vi "GetDeviceSubsetForDeployment.vi"(7 "num":i32=2, 8 "error in (no error)":errorcluster, 9 "i":i32, 10 "DeviceList":T1[](array[typedef])) -> (0 "Error Out":errorcluster, 2 "subarray":T1[](array[typedef]))   [LabVIEW 2016]
uses:
  <vilib>/addons/InsightCM/MessageBus/MessageLibrary/SysCfgDeployer/controls/SysCfgDeployPackageRequestBody.ctl
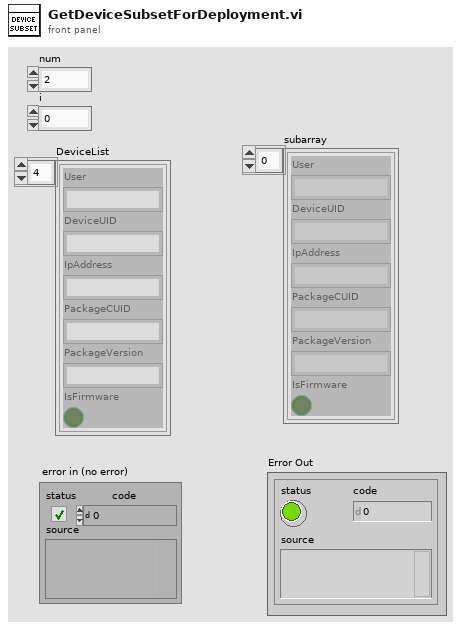
[diagram p1: front panel]
types:
  T1 = typedef "SysCfgDeployPackageRequestBody.ctl" = cluster{"User":string, "DeviceUID":string, "IpAddress":string, "PackageCUID":string, "PackageVersion":string, "IsFirmware":bool}
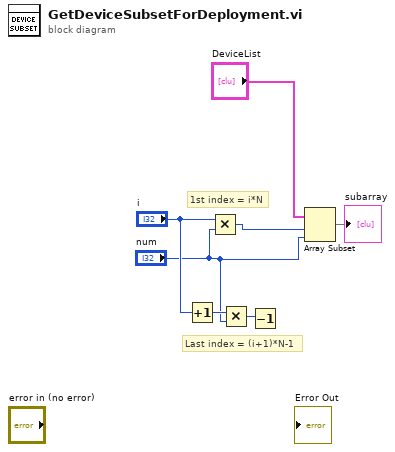
[diagram p0: block diagram]
diagram:
  # "1st index = i*N"
  # "Last index = (i+1)*N-1"
  n1 = Increment(x="i") -> (x+1=w5:i32)
  n2 = Multiply(x="i", y="num") -> (x*y=w2:i32)
  n3 = Multiply(x=w5, y="num") -> (x*y=w4:i32)
  n4 = Decrement(x=w4) -> ()  [unwired: 1 out]
  n5 = Array Subset(array="DeviceList", index=w2, length="num") -> (→"subarray":T1[])
